vi "Instr_SetPrivateData.vi"(8 "error in (no error)":errorcluster, 11 "SupplyControl in":refnum<class "SupplyControl.lvclass">) -> (0 "error out":errorcluster, 3 "SupplyControl out":refnum<class "SupplyControl.lvclass">)   [LabVIEW 2013, in "SupplyControl.lvclass"]
uses:
  SupplyControl.lvclass
  InstrControl.lvclass
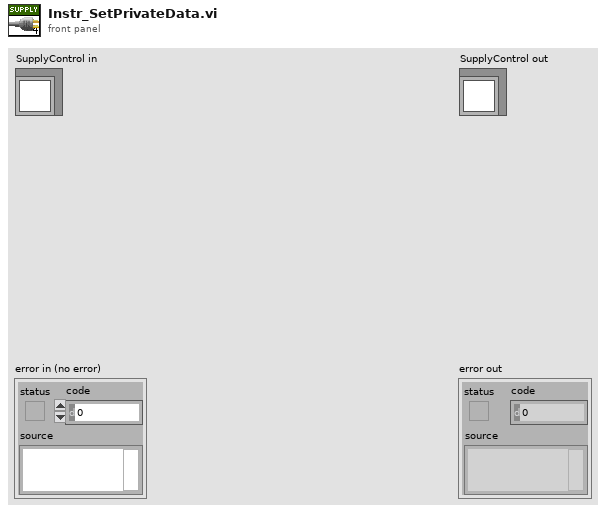
[diagram p1: front panel]
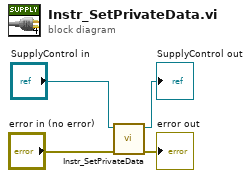
[diagram p0: block diagram]
diagram:
  n1 = call-parent "Instr_SetPrivateData.vi"("error in (no error)"="error in (no error)", "InstrControl in"="SupplyControl in") -> ("error out"=→"error out":errorcluster, "InstrControl out"=→"SupplyControl out":refnum<class "SupplyControl.lvclass">)  [unwired: 8 in]
